vi "Delete Directory.vi"(8 "error in (no error)":errorcluster caption="错误输入（无错误）", 9 "recycle":i32(ring)=2 items=["DeletePermanently"=2, "SendToRecycleBin"=3], 10 "Path":path, 11 "FileSystem 输入":refnum<class "FileSystem.lvclass"> caption="DNL_LabVIEW Object in") -> (0 "error out":errorcluster caption="错误输出", 3 "FileSystem 输出":refnum<class "FileSystem.lvclass"> caption="DNL_LabVIEW Object out")   [LabVIEW 2012, in "FileSystem.lvclass"]
uses:
  FileSystem.lvclass
  FileSystem.lvclass/FileSystem.ctl
  Microsoft.VisualBasic
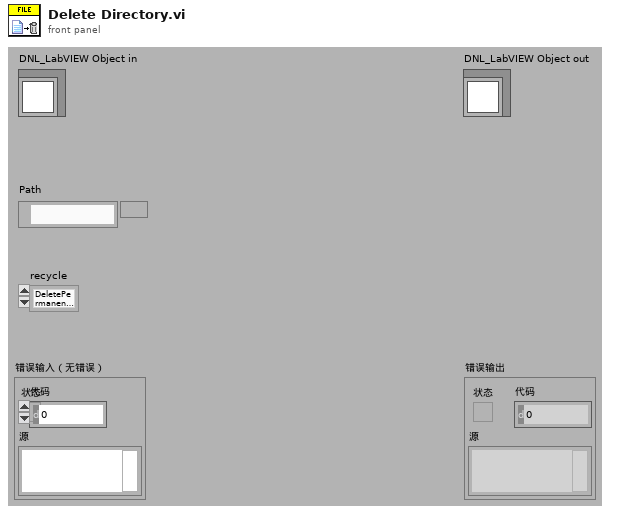
[diagram p1: front panel]
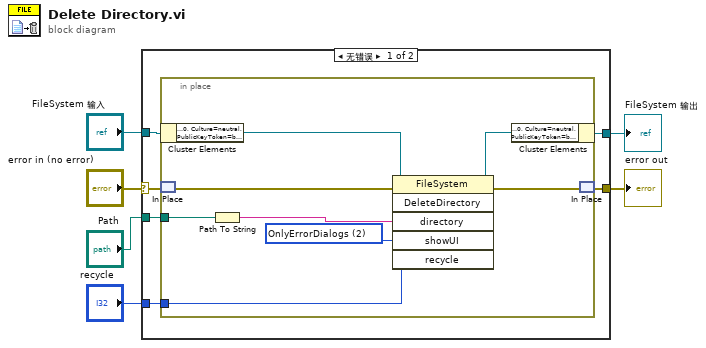
[diagram p0: block diagram]
diagram:
  n1 = case shown="无错误" "error in (no error)" {
    selector: "error in (no error)" -> [w10 w22]
    tunnel: [w9 w22] -> w5
    tunnel: [w11 w21] -> w3
    tunnel: "FileSystem 输入" -> [w12 w21]
    tunnel: "Path" -> [w8 _]
    tunnel: "recycle" -> [w7 _]
    frame No Error {
      n2 = in-place {
        in-place-border: w8 -> [w17]
        in-place-border: w7 -> [w15]
        w18 = 2 items=["OnlyErrorDialogs"=2, "AllDialogs"=3] ("showUI")
        n3 = in-place-cluster #1(w12) -> ("FileSystem"=w20:refnum<k24>)
        n4 = in-place-match #2(w10) -> (w13:errorcluster)
        n5 = Path To String(path=w17) -> (string=w16:string)
        n6 = invoke class="FileSystem" method="DeleteDirectory"(reference=w20, error in=w13, "directory"=w16, "showUI"=w18, "recycle"=w15) -> (reference out=w19:refnum<k24>, error out=w14:errorcluster)  [unwired: 1 in, 4 out]
        n7 = in-place-cluster #1("FileSystem"=w19) -> (w11:refnum<class "FileSystem.lvclass">)
        n8 = in-place-match #2(w14) -> (w9:errorcluster)
      }
    }
    frame Error {
    }
  }
  "error out" <- w5
  "FileSystem 输出" <- w3
